vi "EventStructureBasedExample_MCA_Program.vi"() -> ()   [LabVIEW 2014]
uses:
  Typedef_MCAControl.ctl
panel:
  out "CoincidenceWindow":i32[](graph)=[25, 24, 24, 25, 21, 20, 26, 14, 28, 16, 21, 16, 13, 16, 18, 19, 18, 19, 18, 25, 24, 25, 35, 34, 27, 38, 48, 50, 60, 58, 61, 58, 56, 49, 36, 30, 41, 36, 18, 24, 22, 20, 21, 20, 14, 13, 23, 32, 30, 16, 26, 27, 15, 22, 19, 25, 20, 18, 24, 29, 24]
  out "Coincidence Counts":dbl=436.94988864142533 format="%.1f"
  in  "ROI Settings":T1={"Signal Min (ns)"=600, "Signal Max (ns)"=660, "Background Min (ns)"=20, "Background Max (ns)"=980}
  in  "TAC Settings":cluster{"Full Scale (ns)":dbl, "# bins":i32}={"Full Scale (ns)"=1000.0, "# bins"=1000} {"# bins" min=1 max=65535 step=1; "Full Scale (ns)" format="%0.2f"}
  in  "Reset":bool
  in  "Pause":bool
  out "Coincidence Signal":cluster{"Axis":dbl[], i32[]}(graph)={"Axis"=array[1001 elements], [7, 16, 30, 17, 28, 21, 19, 13, 24, 22, 15, 20, 27, 16, 20, 21, 23, 20, 21, 23, 19, 14, 19, 19, 24, 14, 23, 15, 21, 24, 16, 22, 16, 25, 21, 15, 20, 23, 18, 24, 27, 25, 30, 22, 22, 18, 17, 13, 13, 21, 17, 25, 21, 24, 14, 20, 14, 18, 20, 21, 18, 18, 20, 14, 26, 15, 17, 27, 18, 20, 25, 32, 26, 18, 16, 18, 22, 16, 19, 18, 15, 24, 15, 21, 19, 30, 25, 14, 21, 24, 19, 25, 24, 24, 20, 19, 20, 12, 18, 13, 17, 21, 16, 19, 15, 17, 24, 17, 26, 17, 25, 25, 15, 25, 21, 24, 17, 22, 18, 21, 15, 25, 18, 19, 25, 15, 20, 17, 18, 23, 18, 21, 24, 22, 21, 16, 30, 10, 20, 18, 21, 20, 30, 17, 24, 30, 27, 14, 18, 18, 18, 20, 27, 25, 23, 24, 19, 20, 13, 19, 20, 24, 15, 16, 25, 21, 17, 26, 20, 22, 19, 18, 25, 26, 23, 24, 30, 26, 22, 14, 20, 25, 20, 18, 27, 11, 22, 19, 17, 25, 22, 22, 14, 34, 32, 22, 14, 20, 21, 22, 23, 17, 28, 28, 14, 17, 16, 21, 21, 9, 26, 14, 18, 17, 24, 19, 19, 17, 26, 14, 13, 32, 15, 23, 19, 14, 24, 26, 18, 24, 29, 21, 21, 14, 22, 17, 11, 26, 27, 20, 14, 18, 14, 21, 17, 24, 18, 22, 18, 26, 20, 19, 22, 18, 18, 17, 25, 23, 22, 27, 22, 18, 20, 24, 23, 21, 24, 15, 20, 28, 19, 20, 16, 23, 13, 22, 18, 20, 23, 18, 23, 6, 19, 10, 16, 13, 18, 25, 16, 21, 17, 27, 19, 17, 20, 21, 25, 21, 15, 11, 18, 22, 15, 16, 20, 22, 21, 24, 24, 17, 13, 15, 22, 24, 20, 9, 14, 6, 23, 22, 21, 21, 15, 23, 17, 18, 22, 20, 24, 26, 18, 15, 27, 18, 20, 12, 24, 19, 15, 24, 22, 12, 18, 16, 22, 22, 17, 20, 21, 13, 17, 21, 17, 16, 12, 12, 10, 20, 31, 24, 18, 15, 23, 24, 26, 32, 25, 19, 22, 17, 22, 19, 25, 26, 16, 18, 21, 19, 21, 23, 23, 15, 16, 17, 22, 20, 23, 26, 25, 28, 22, 24, 14, 25, 17, 20, 24, 18, 19, 11, 22, 24, 26, 13, 24, 21, 17, 23, 17, 16, 24, 18, 21, 13, 23, 23, 29, 23, 21, 14, 20, 18, 16, 19, 26, 17, 19, 19, 18, 26, 13, 16, 20, 18, 18, 11, 23, 18, 16, 13, 24, 18, 17, 14, 21, 11, 19, 36, 19, 25, 16, 21, 24, 23, 20, 22, 19, 22, 21, 14, 15, 19, 30, 14, 27, 25, 23, 14, 22, 14, 24, 17, 27, 25, 24, 18, 31, 22, 21, 19, 23, 17, 23, 23, 24, 19, 18, 18, 23, 19, 20, 10, 19, 22, 27, 23, 23, 19, 19, 29, 23, 18, 27, 19, 19, 23, 21, 19, 12, 19, 23, 20, 22, 19, 12, 15, 23, 19, 16, 15, 18, 22, 23, 31, 22, 31, 18, 28, 29, 14, 21, 16, 19, 19, 13, 19, 15, 26, 27, 22, 24, 25, 22, 18, 26, 17, 21, 22, 27, 23, 16, 15, 17, 20, 21, 32, 21, 28, 22, 22, 30, 19, 19, 22, 19, 18, 28, 25, 26, 28, 16, 29, 27, 16, 23, 18, 18, 18, 21, 21, 11, 15, 19, 18, 18, 21, 23, 22, 18, 17, 16, 25, 21, 22, 13, 17, 20, 17, 25, 30, 25, 24, 24, 25, 21, 20, 26, 14, 28, 16, 21, 16, 13, 16, 18, 19, 18, 19, 18, 25, 24, 25, 35, 34, 27, 38, 48, 50, 60, 58, 61, 58, 56, 49, 36, 30, 41, 36, 18, 24, 22, 20, 21, 20, 14, 13, 23, 32, 30, 16, 26, 27, 15, 22, 19, 25, 20, 18, 24, 29, 24, 25, 22, 18, 17, 15, 21, 16, 21, 22, 23, 21, 26, 25, 18, 17, 25, 22, 21, 18, 35, 18, 25, 30, 17, 18, 21, 13, 21, 19, 16, 22, 20, 23, 19, 16, 19, 23, 25, 18, 23, 10, 24, 19, 17, 22, 21, 27, 17, 21, 13, 12, 24, 14, 15, 25, 18, 13, 22, 20, 21, 13, 17, 16, 20, 23, 19, 30, 12, 17, 16, 24, 21, 20, 26, 20, 24, 10, 26, 17, 23, 22, 22, 18, 29, 20, 29, 27, 20, 21, 20, 20, 24, 17, 12, 17, 20, 24, 19, 20, 22, 19, 16, 27, 21, 16, 20, 16, 21, 20, 14, 19, 29, 29, 24, 21, 19, 25, 12, 22, 17, 19, 20, 16, 21, 13, 17, 18, 27, 24, 18, 16, 25, 20, 11, 19, 20, 19, 30, 19, 29, 18, 18, 22, 18, 18, 12, 27, 14, 36, 21, 10, 16, 22, 22, 23, 23, 21, 16, 24, 20, 18, 19, 15, 20, 18, 23, 6, 17, 28, 21, 21, 20, 18, 18, 18, 18, 26, 18, 17, 16, 24, 15, 19, 16, 13, 24, 18, 22, 19, 12, 21, 24, 6, 16, 28, 18, 22, 18, 17, 21, 24, 24, 26, 28, 23, 19, 27, 18, 16, 20, 29, 26, 31, 26, 25, 25, 18, 19, 22, 23, 18, 15, 23, 22, 20, 22, 24, 20, 29, 26, 22, 32, 27, 16, 20, 17, 18, 19, 17, 27, 22, 19, 17, 13, 27, 21, 27, 23, 21, 29, 18, 18, 21, 22, 19, 18, 14, 19, 24, 19, 22, 20, 15, 20, 21, 26, 24, 22, 25, 23, 14, 23, 21, 16, 11, 21, 22, 20, 30, 21, 18, 13, 20, 26, 31, 18, 20, 22, 21, 19, 29, 23, 13, 30, 20, 20, 19, 15, 23, 18, 18, 24, 19, 29, 21, 19, 18, 18, 24, 19, 17, 15, 20, 10, 17, 16, 14, 19, 11, 24, 16, 22, 20, 15, 27, 28, 24, 23, 21, 15, 11, 27, 26, 14, 22, 18, 23, 12, 21, 18]}
  out "Total Time (s)":dbl=60.5
  out "Delta Time (s)":dbl=0.001
  out "error out":errorcluster
  in  "Update Rate (Hz)":u32=10 min=1 max=1000 step=1
  in  "Stop Button":bool
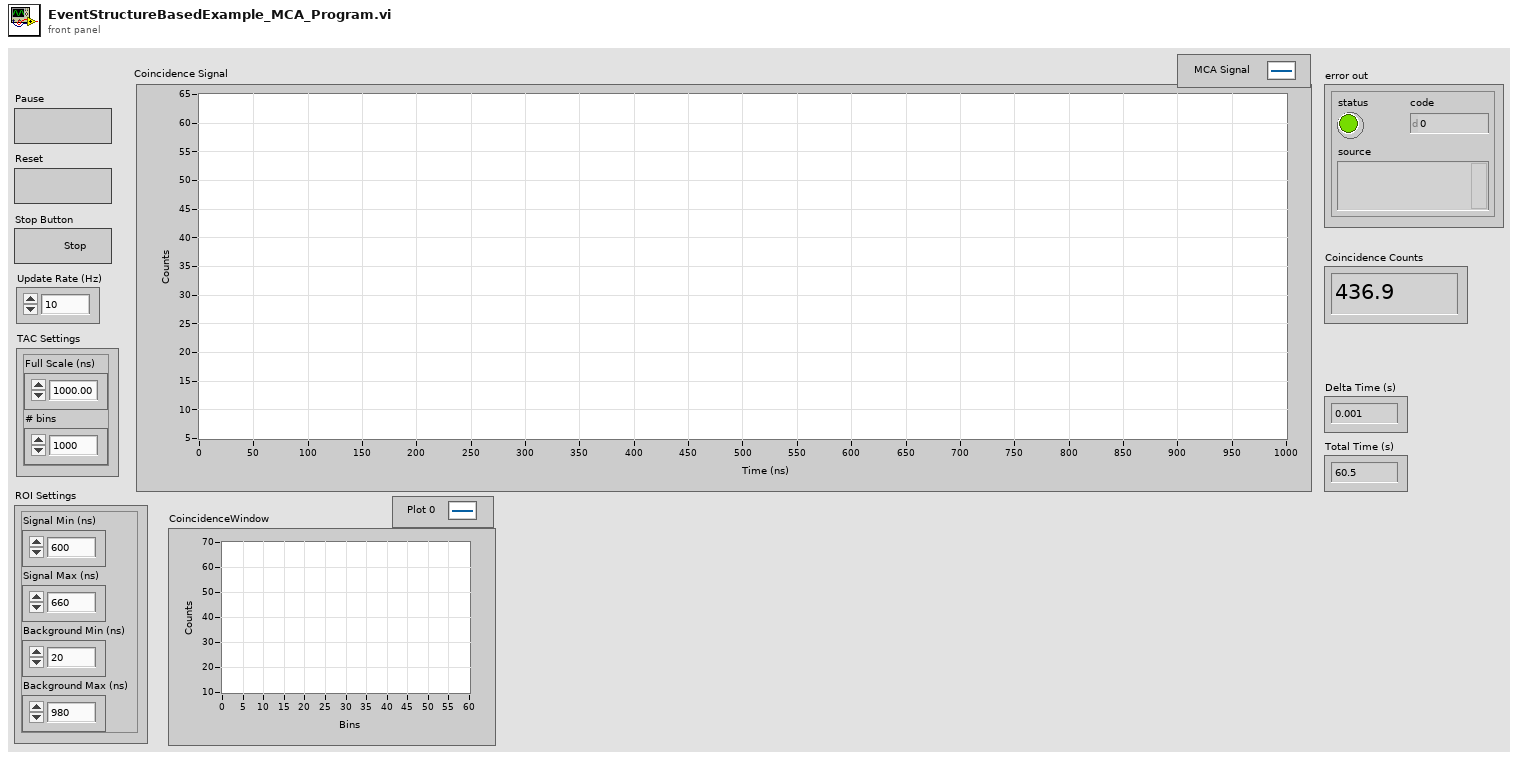
[diagram p1: front panel]
types:
  T1 = cluster{"Signal Min (ns)":i32, "Signal Max (ns)":i32, "Background Min (ns)":i32, "Background Max (ns)":i32}
  T2 = enum16{"Start Running", "Stop Running", "Check State"}
  T3 = typedef "Typedef_MCAControl.ctl" = enum16{"Start", "Check", "Pause", "Unpause", "Update Settings", "Reset", "Stop"}
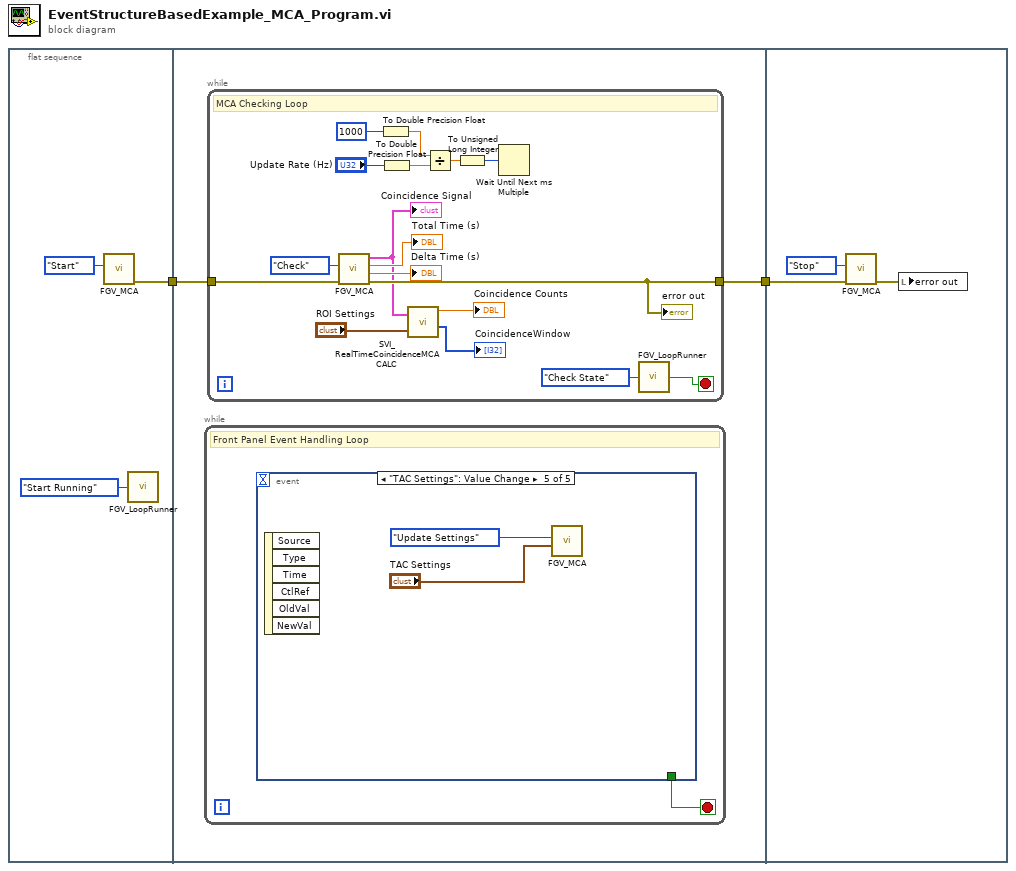
[diagram p0: block diagram]
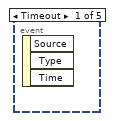
[diagram p2: hidden frame]
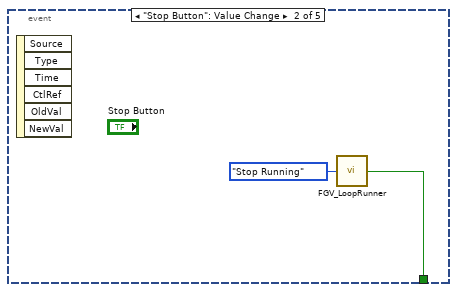
[diagram p3: hidden frame]
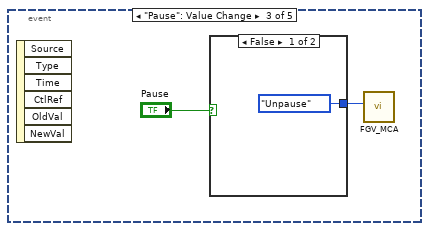
[diagram p4: hidden frame]
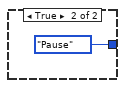
[diagram p5: hidden frame]
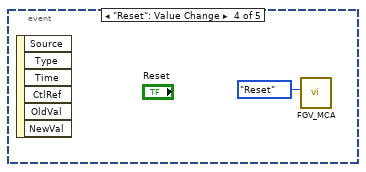
[diagram p6: hidden frame]
diagram:
  n1 = flat-sequence {
    tunnel: [w3] -> w2
    tunnel: w2 -> [w7]
    tunnel: [w6] -> w1
    tunnel: w1 -> [w36]
    frame #0 {
      n2 = call "FGV_MCA.vi"("MCA Action"=Typedef_MCAControl."Start") -> ("error out"=w3:errorcluster)  [unwired: 6 in, 4 out]
      n3 = call "FGV_LoopRunner.vi"("Loop Controller"=T2."Start Running") -> ()  [unwired: 1 out]
    }
    frame #1 {
      n4 = while {
        stop <- w25 stop-if-true
        # "Front Panel Event Handling Loop"
        n5 = event shown="[4] \"TAC Settings\": Value Change" {
          selector: _ -> [_ _ _ _ _]
          dyn-events: _ -> [_ _ _ _ _]
          timeout: _ -> [_ _ _ _ _]
          tunnel: [_ w26 _ _ _] -> w25
          event Timeout {
            n6 = event-data() -> ()  [unwired: 1 in, 3 out]
          }
          event "Stop Button": Value Change {
            n7 = event-data() -> ()  [unwired: 1 in, 6 out]
            n8 = call "FGV_LoopRunner.vi"("Loop Controller"=T2."Stop Running") -> ("Stop Loops"=w26:bool)
          }
          event "Pause": Value Change {
            n9 = event-data() -> ()  [unwired: 1 in, 6 out]
            n10 = case shown="False" "Pause" {
              tunnel: [Typedef_MCAControl."Unpause" ("MCA Action") Typedef_MCAControl."Pause" ("MCA Action")] -> w28
              frame False {
              }
              frame True {
              }
            }
            n11 = call "FGV_MCA.vi"("MCA Action"=w28) -> ()  [unwired: 6 in, 5 out]
          }
          event "Reset": Value Change {
            n12 = event-data() -> ()  [unwired: 1 in, 6 out]
            n13 = call "FGV_MCA.vi"("MCA Action"=Typedef_MCAControl."Reset") -> ()  [unwired: 6 in, 5 out]
          }
          event "TAC Settings": Value Change {
            n14 = event-data() -> ()  [unwired: 1 in, 6 out]
            n15 = call "FGV_MCA.vi"("TAC Settings"="TAC Settings", "MCA Action"=Typedef_MCAControl."Update Settings") -> ()  [unwired: 5 in, 5 out]
          }
        }
      }
      n16 = while {
        tunnel: w7 -> [w15]
        tunnel: [w14] -> w6
        stop <- w24 stop-if-true
        # "MCA Checking Loop"
        n17 = call "FGV_MCA.vi"("Error In"=w15, "MCA Action"=Typedef_MCAControl."Check") -> ("error out"=w14:errorcluster, "Delta Time (s)"=→"Delta Time (s)":dbl, "Total Time (s)"=→"Total Time (s)":dbl, "Coincidence Signal"=w11:cluster{"Axis":dbl[], i32[]})  [unwired: 5 in, 1 out]
        "error out" <- w14
        "Coincidence Signal" <- w11
        n18 = To Double Precision Float(number=u32 1000 ("x")) -> (double precision float=w16:dbl)
        n19 = To Double Precision Float(number="Update Rate (Hz)") -> (double precision float=w17:dbl)
        n20 = call "SVI_RealTimeCoincidenceMCACALC.vi"("Coincidence Signal"=w11, "ROI Settings"="ROI Settings") -> ("Coincidence Counts"=→"Coincidence Counts":dbl, "CoincidenceWindow"=→"CoincidenceWindow":i32[])  [unwired: 2 out]
        n21 = Divide(x=w16, y=w17) -> (x/y=w19:dbl)
        n22 = To Unsigned Long Integer(number=w19) -> (unsigned 32bit integer=w18:u32)
        n23 = Wait Until Next ms Multiple(millisecond multiple=w18) -> ()  [unwired: 1 out]
        n24 = call "FGV_LoopRunner.vi"("Loop Controller"=T2."Check State") -> ("Stop Loops"=w24:bool)
      }
    }
    frame #2 {
      n25 = call "FGV_MCA.vi"("Error In"=w36, "MCA Action"=Typedef_MCAControl."Stop") -> ("error out"=w35:errorcluster)  [unwired: 5 in, 4 out]
      n26 = local write "error out"(w35) -> ()
    }
  }
